vi "SIM limit signal.vi"   [LabVIEW 2010]
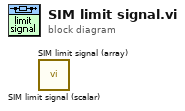
[diagram p0: block diagram]
diagram:
  n1 = call "SIM limit signal (scalar).vi"() -> ()  [unwired: 10 in, 2 out]
  n2 = call "SIM limit signal (array).vi"() -> ()  [unwired: 10 in, 2 out]
